vi "Check First Timestamp.vi"(8 "error in (no error)":errorcluster, 11 "Waveform Generator in":refnum<class "Waveform Generator.lvclass">) -> (0 "error out":errorcluster, 2 "Is First":bool=TRUE, 3 "Waveform Generator out":refnum<class "Waveform Generator.lvclass">)   [LabVIEW 2015, in "Waveform Generator.lvclass"]
uses:
  Waveform Generator.lvclass
  Waveform Generator.lvclass/Waveform Generator.ctl
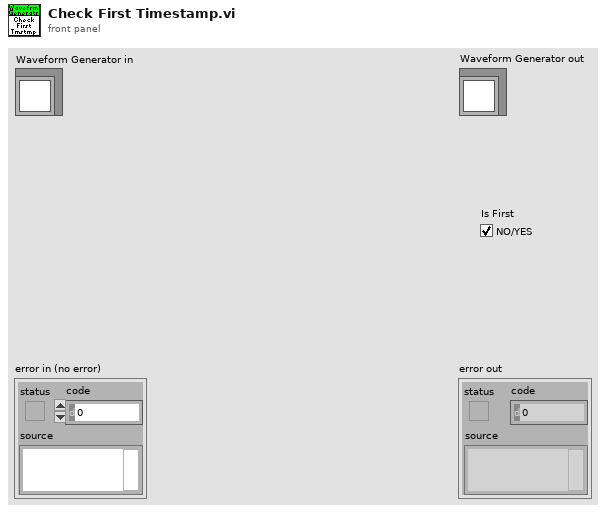
[diagram p1: front panel]
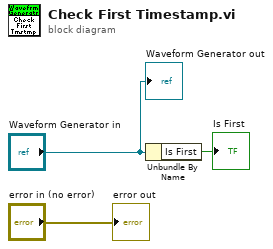
[diagram p0: block diagram]
diagram:
  n1 = Unbundle By Name("Waveform Generator in") -> ("Is First"=→"Is First":bool)
  "error out" <- "error in (no error)"
  "Waveform Generator out" <- "Waveform Generator in"
